vi "S2C_VLFT10_Proc_ClearFornaxMsgs.vi"(8 "Error In":errorcluster, 11 "ClearMsg":string) -> (0 "Error Out":errorcluster)   [LabVIEW 2015]
uses:
  Fornax/VIs/S2C_FORNAX_Proc_Globals.vi
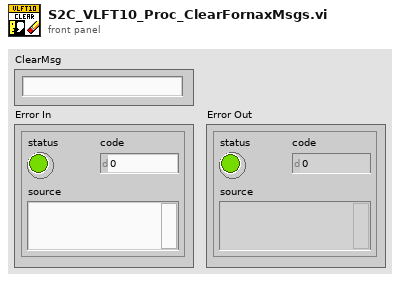
[diagram p1: front panel]
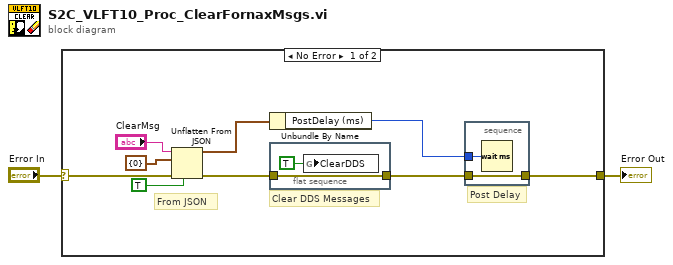
[diagram p0: block diagram]
diagram:
  n1 = case shown="No Error" "Error In" {
    selector: "Error In" -> [w11 w16]
    tunnel: [w5 w16] -> w1
    frame No Error {
      # "Clear DDS Messages"
      # "Post Delay"
      # "From JSON"
      n2 = Unflatten From JSON(JSON string="ClearMsg", type and defaults=cluster{"PostDelay (ms)":i32} {"PostDelay (ms)"=0}, default null elements? (F)=TRUE, error in (no error)=w11) -> (value=w7:cluster{"PostDelay (ms)":i32}, error out=w4:errorcluster)  [unwired: 3 in]
      n3 = Unbundle By Name(w7) -> ("PostDelay (ms)"=w6:i32)
      n4 = flat-sequence {
        tunnel: w4 -> [w12]
        tunnel: [w12] -> w3
        frame #0 {
          n5 = global write "S2C_FORNAX_Proc_Globals.vi" "ClearDDS"(TRUE ("ClearDDS")) -> ()
        }
      }
      n6 = stacked-sequence {
        tunnel: w3 -> [w15]
        tunnel: [w15] -> w5
        tunnel: w6 -> [w14]
        frame #0 {
          n7 = Wait (ms)(milliseconds to wait=w14) -> ()  [unwired: 1 out]
        }
      }
    }
    frame Error {
    }
  }
  "Error Out" <- w1
